vi "Expand Structure into Triclinic.vi"(6 "Max # of atoms":i32=9999999, 8 "New Lattice Vector c":dbl[](array[numeric])=[0.0, 0.0, 6.0], 9 "New Lattice Vector b":dbl[](array[numeric])=[0.0, 6.0, 0.0], 10 "New Lattice Vector a":dbl[](array[numeric])=[6.0, 0.0, 0.0], 11 "Primitive Unit Cell":T1={"Structure Name"="CdTe", "Lattice vector a"=[6.615785553057252, 0.0, 0.0], "Lattice vector b"=[0.0, 6.615785553057252, 0.0], "Lattice vector c"=[0.0, 0.0, 6.615785553057252], "Atoms Array"=[{"Atom Name"="Cd", "Positions (Direct)"=[[0.0, 0.0, 0.0], [0.0, 0.5, 0.5], [0.5, 0.0, 0.5], [0.5, 0.5, 0.0]], "Positions (Cartesian)"=[[0.0, 0.0, 0.0], [0.0, 3.307892776528626, 3.307892776528626], [3.307892776528626, 0.0, 3.307892776528626], [3.307892776528626, 3.307892776528626, 0.0]]}, {"Atom Name"="Te", "Positions (Direct)"=[[0.25, 0.25, 0.25], [0.75, 0.75, 0.25], [0.75, 0.25, 0.75], [0.25, 0.75, 0.75]], "Positions (Cartesian)"=[[1.653946388264313, 1.653946388264313, 1.653946388264313], [4.96183916479294, 4.96183916479294, 1.653946388264313], [4.96183916479294, 1.653946388264313, 4.96183916479294], [1.653946388264313, 4.96183916479294, 4.96183916479294]]}], "# of atoms"=8}) -> (3 "Expanded Structure":T1={"Structure Name"="Reduced CdTe Expanded to Box", "Lattice vector a"=[6.0, 0.0, 0.0], "Lattice vector b"=[0.0, 6.0, 0.0], "Lattice vector c"=[0.0, 0.0, 6.0], "Atoms Array"=[{"Atom Name"="Cd", "Positions (Direct)"=[[0.00016666666666666666, 0.00016666666666666666, 0.16881746031746028], [0.00016666666666666666, 0.04433375914924137, 0.9472432736655599], [0.00016666666666666666, 0.7785924800147661, 0.12465036783488567], [0.00016666666666666666, 0.8227595724973409, 0.9030761811829852], [0.5514821294214376, 0.41146311958200377, 0.5359468207502227]], "Positions (Cartesian)"=[[0.0, 0.0, 1.0119047619047619], [0.0, 0.2650025548954482, 5.6824596419933595], [0.0, 4.670554880088597, 0.7469022070093141], [0.0, 4.935557434984045, 5.417457087097911], [3.307892776528626, 2.4677787174920227, 3.2146809245013364]]}, {"Atom Name"="Te", "Positions (Direct)"=[[0.2758243980440521, 0.022250212907954016, 0.5580303669915101], [0.2758243980440521, 0.8006760262560535, 0.5138632745089352], [0.8271398607988233, 0.3893795733407164, 0.14673391407617298], [0.8271398607988233, 0.43354666582329104, 0.9251597274242727]], "Positions (Cartesian)"=[[1.653946388264313, 0.1325012774477241, 3.3471822019490607], [1.653946388264313, 4.803056157536321, 3.0821796470536116], [4.96183916479294, 2.3352774400442984, 0.879403484457038], [4.96183916479294, 2.6002799949397466, 5.549958364545636]]}], "# of atoms"=9} {"Atoms Array"."Positions (Cartesian)" format="%#_4f"; "Atoms Array"."Positions (Direct)" format="%#_4f"})   [LabVIEW 2010]
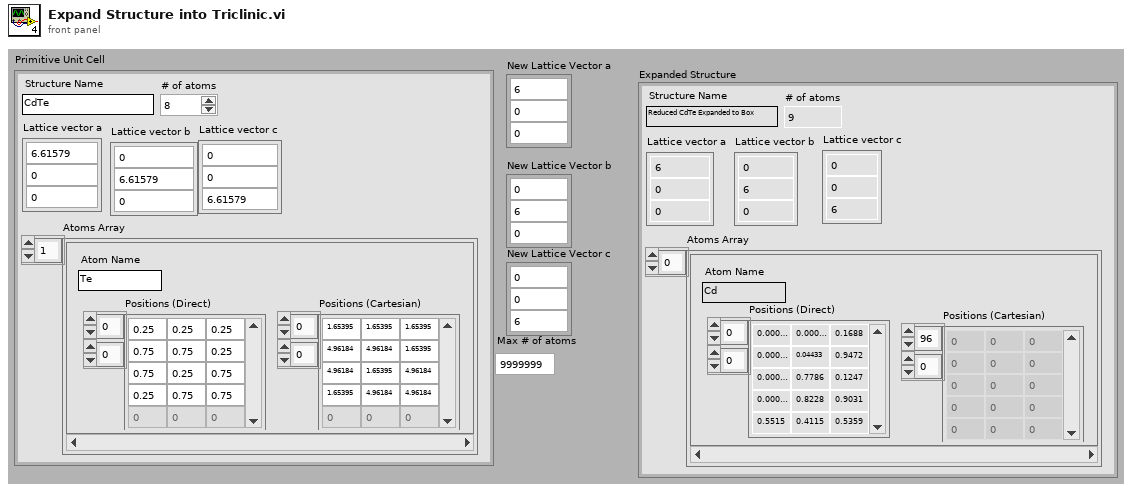
[diagram p1: front panel]
types:
  T1 = cluster{"Structure Name":string, "Lattice vector a":dbl[], "Lattice vector b":dbl[], "Lattice vector c":dbl[], "Atoms Array":cluster{"Atom Name":string, "Positions (Direct)":dbl[][], "Positions (Cartesian)":dbl[][]}[], "# of atoms":i32}
  T2 = cluster{"Z Min":dbl, dbl, "Z Min":dbl, dbl, "Z Min":dbl, dbl}
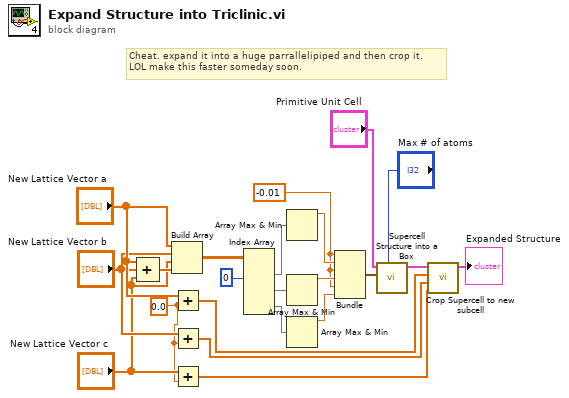
[diagram p0: block diagram]
diagram:
  w2 = -0.01 ("Z Min")
  w3 = 0.0 ("Z Min")
  # "Cheat. expand it into a huge parrallelipiped and then crop it.\nLOL make this faster someday soon."
  n1 = Compound Arithmetic op=ADD("New Lattice Vector a", "New Lattice Vector b", "New Lattice Vector c") -> (w14:dbl[])
  n2 = Build Array("New Lattice Vector a", "New Lattice Vector b", "New Lattice Vector c", w14) -> (w21:dbl[][])
  n3 = Add(x="New Lattice Vector a", y=w3) -> (x+y=w10:dbl[])
  n4 = Add(x="New Lattice Vector b", y=w3) -> (x+y=w7:dbl[])
  n5 = Add(x="New Lattice Vector c", y=w3) -> (x+y=w6:dbl[])
  n6 = Index Array(array=w21, index (col) #1=0 ("disabled index (col)")) -> (element #1=w19:dbl[], element #2=w18:dbl[], element #3=w17:dbl[])  [unwired: 5 in]
  n7 = Array Max & Min(array=w19) -> (max value=w4:dbl)  [unwired: 3 out]
  n8 = Array Max & Min(array=w18) -> (max value=w16:dbl)  [unwired: 3 out]
  n9 = Array Max & Min(array=w17) -> (max value=w15:dbl)  [unwired: 3 out]
  n10 = Bundle("Z Min"=w2, w4, "Z Min"=w2, w16, "Z Min"=w2, w15) -> (w1:T2)  [unwired: 1 in]
  n11 = call "Supercell Structure into a Box.vi"("Max # of atoms"="Max # of atoms", "Draw Box"=w1, "Subcrystal"="Primitive Unit Cell") -> ("Expanded cubic Structure"=w22:T1)  [unwired: 6 in, 2 out]
  n12 = call "Crop Supercell to new subcell.vi"("New Lattice Vector c"=w6, "New Lattice Vector b"=w7, "New Lattice Vector a"=w10, "Supercell Structure"=w22) -> ("Reduced Structure"=→"Expanded Structure":T1)  [unwired: 7 in]
